vi "PAT Device Software 1.6.vi"() -> ()   [LabVIEW 2018]
uses:
  <vilib>/Utility/error.llb/DialogType.ctl
  <vilib>/DAQmx/write.llb/DAQmx Write (Analog 1D DBL NChan 1Samp).vi
  <vilib>/DAQmx/read.llb/DAQmx Read (Analog 1D DBL NChan 1Samp).vi
  <vilib>/DAQmx/write.llb/DAQmx Write (Analog DBL 1Chan 1Samp).vi
  <vilib>/Instr/_visa.llb/VISA Configure Serial Port (Instr).vi
  <vilib>/DAQmx/create/channels.llb/DAQmx Create Channel (AO-Voltage-Basic).vi
  <vilib>/DAQmx/create/channels.llb/DAQmx Create Channel (AI-Voltage-Basic).vi
  <vilib>/DAQmx/configure/timing.llb/DAQmx Timing (Sample Clock).vi
  <vilib>/DAQmx/miscellaneous.llb/DAQmx Fill In Error Info.vi
panel:
  out "Load Preset":bool
  in  "command line":string="cmd /c \"C:\\Program Files (x86)\\QTenki\\usbtenkiget.exe\" -s E13367 -i 0,1,2"
  in  "Test Length":i32=15
  in  "Minute Volume":dbl format="%#_13g"
  out "CV2 Voltage":dbl format="%#_13g"
  out "CV1 Voltage":dbl format="%#_13g"
  in  "In Progress":bool
  out "Total Test Time":i32
  in  "Test Buffer Duration":i32=10
  in  "Motor Control":bool
  out "Corrected Voltage":dbl=3.0 format="%#_13g"
  out "Rotation Time":dbl format="%#_3g"
  out "Error Ratio":dbl format="%#_13g"
  out "Reference Voltage":dbl=3.001413381851861 format="%0.2f"
  out "Hit Recorded":bool
  in  "CV2 Output":tag="Dev1/ao0"
  in  "CV1 Output":tag="Dev1/ao1"
  in  "Motor Output":tag="Dev2/ao0"
  in  "Hall Sensor Channel":tag="Dev2/ai7"
  in  "O2 Channel":tag="Dev2/ai6"
  in  "P2 Channel":tag="Dev2/ai4"
  in  "Relay Port":refnum<visa-resource-name>="COM13"
  in  "Sample Rate":i32=10
  in  "CV2 Channel":tag="Dev1/ai6"
  in  "CV1 Channel":tag="Dev1/ai3"
  in  "P1 Channel":tag="Dev1/ai5"
  out "Stop Test":bool=TRUE
  out "Is PAT Test?":bool
  in  "Test Begin":bool
  out "Test Duration":i32
  out "Current Test":string
  out "Test Underway":i32
  out "Number of tests":i32=4
  out "Test List":i16[](array[numeric])=[1, 1, 1, 1, 0, 0]
  out "error out 3":errorcluster
  in  "error in 2":errorcluster
  out "error out 2":errorcluster
  in  "error in":errorcluster
  out "error out":errorcluster
  in  "error in (no error)":errorcluster
  in  "Tab Control":enum32{"PAT Test", "Manual Control"}(tab)
  out "PAT Test Readings":T1 {"B40 S" scale=0.0..100.0; "B15 S" scale=0.0..100.0; "Ex70 S" scale=0.0..100.0; "Ex30 S" scale=0.0..100.0; "In70 S" scale=0.0..100.0; "B15 M" format="%#.2g"; "B40 M" format="%#.2g"; "Ex70 M" format="%#.2g"; "Ex30 M" format="%#.2g"; "In70 M" format="%#.2g"; "In30 S" scale=0.0..100.0; "In30 M" format="%#.2g"}
  out "Status":string="Status"
  out "Time":string="Time (s)"
  out "Limit":string="Limit"
  out "Comp":string="Comp"
  out "Units":string="Units"
  out "Measured":string="Measured"
  out "Test Name":string="Test Name"
  out "String 22":string="-0.8"
  out "String 24":string="0.8"
  out "String 23":string="-2.0"
  out "String 26":string="26"
  out "String 25":string="2.0"
  out "String 27":string="89"
  out "String 15":string=">="
  out "String 17":string="<="
  out "String 16":string=">="
  out "String 19":string=">="
  out "String 18":string="<="
  out "String 20":string=">="
  out "In H2O":string="in H2O"
  out "In H2O":string="in H2O"
  out "In H2O":string="in H2O"
  out "%O2":string="% O2"
  out "In H2O":string="in H2O"
  out "%O2":string="% O2"
  out "Inhalation 30lpm":string="Inhalation (30lpm)"
  out "Exhalation 30lpm":string="Exhalation (30lpm)"
  out "Inhalation 70lpm":string="Inhalation (70lpm)"
  out "Breathing 15kft":string="Breathing (15kft)"
  out "Exhalation 70lpm":string="Exhalation (70lpm)"
  out "Breathing 40kft":string="Breathing (40kft)"
  in  "Start PAT Test":bool
  in  "Stop PAT Test":bool
  out "Test Status:":string
  in  "Results File Location:":path=path "C:/"
  in  "PAT Test Fields":T2={"Operator:"="", "Pull Test Date:"="", "Manufacture Date:"="", "Cure Date:"="", "Production Order No.:"="", "Production Lot:"="", "No. Masks in Lot:"="", "Comments:"="", "Test Date:"="24 Jan 2019", "Test Time:"="11:23:54", "Test Selection Radio Array"=[TRUE, TRUE, TRUE, TRUE, FALSE, FALSE], "Test Parameters:"=enum."Quick Test", "F2 Leakage"=0.0}
  out "Ambient Pressure:":dbl format="%#.2g"
  out "Ambient Temp.:":dbl format="%#.2g"
  out "Ambient Humidity:":dbl format="%#.2g"
  in  "Preset Directory:":path=path "C:/"
  in  "MC Fields":T3={"Test Date:"="24 Jan 2019", "Test Time:"="11:23:54", "Operator:"="", "Production Order No.:"="", "Production Lot:"="", "No. Masks in Lot:"="", "Test Duration"=0, "Presets in Directory:"=0, "MC Test Length"=enum."Run Continuously", "Current Preset:"="Breathing Test 2.ini", "Preset Save"=FALSE}
  in  "MC Instrumentation":T4={"SV1"=FALSE, "SV2"=FALSE, "SV3"=FALSE, "SV4"=FALSE, "SV5"=FALSE, "SV6"=FALSE, "SV7"=FALSE, "SV8"=FALSE, "SV9"=FALSE, "M1"=FALSE, "MP1"=FALSE, "MP2"=FALSE, "CV1"=FALSE, "CV2"=FALSE, "CV1 Flow Rate:"=0.0, "CV2 Flow Rate:"=0.0, "P2 Pressure:"=0.0, "O2 Concentration:"=0.0, "Motor Speed:"=15.0, "F2 Leakage"=0.0, "P1 Pressure:"=0.0} {"P1 Pressure:" format="%#.2g"; "P2 Pressure:" format="%#.2g"; "O2 Concentration:" format="%#.2g"; "Motor Speed:" min=0.0 max=17.5 step=0.25 format="%#.2g"; "F2 Leakage" min=0.0 max=100.0 step=1.0; "CV2 Flow Rate:" min=0.0 max=100.0 format="%#.2g"; "CV1 Flow Rate:" min=0.0 max=5.0 step=0.5}
  in  "Start Custom Test":bool
  in  "Stop Custom Test":bool
  # "ccm"
  # "s"
  # "Pamb"
  # "Tamb"
  # "Hamb"
  # "in H2O"
  # "°C"
  # "%"
  # "O2"
  # "P"
  # "P"
  # "O2 Supply"
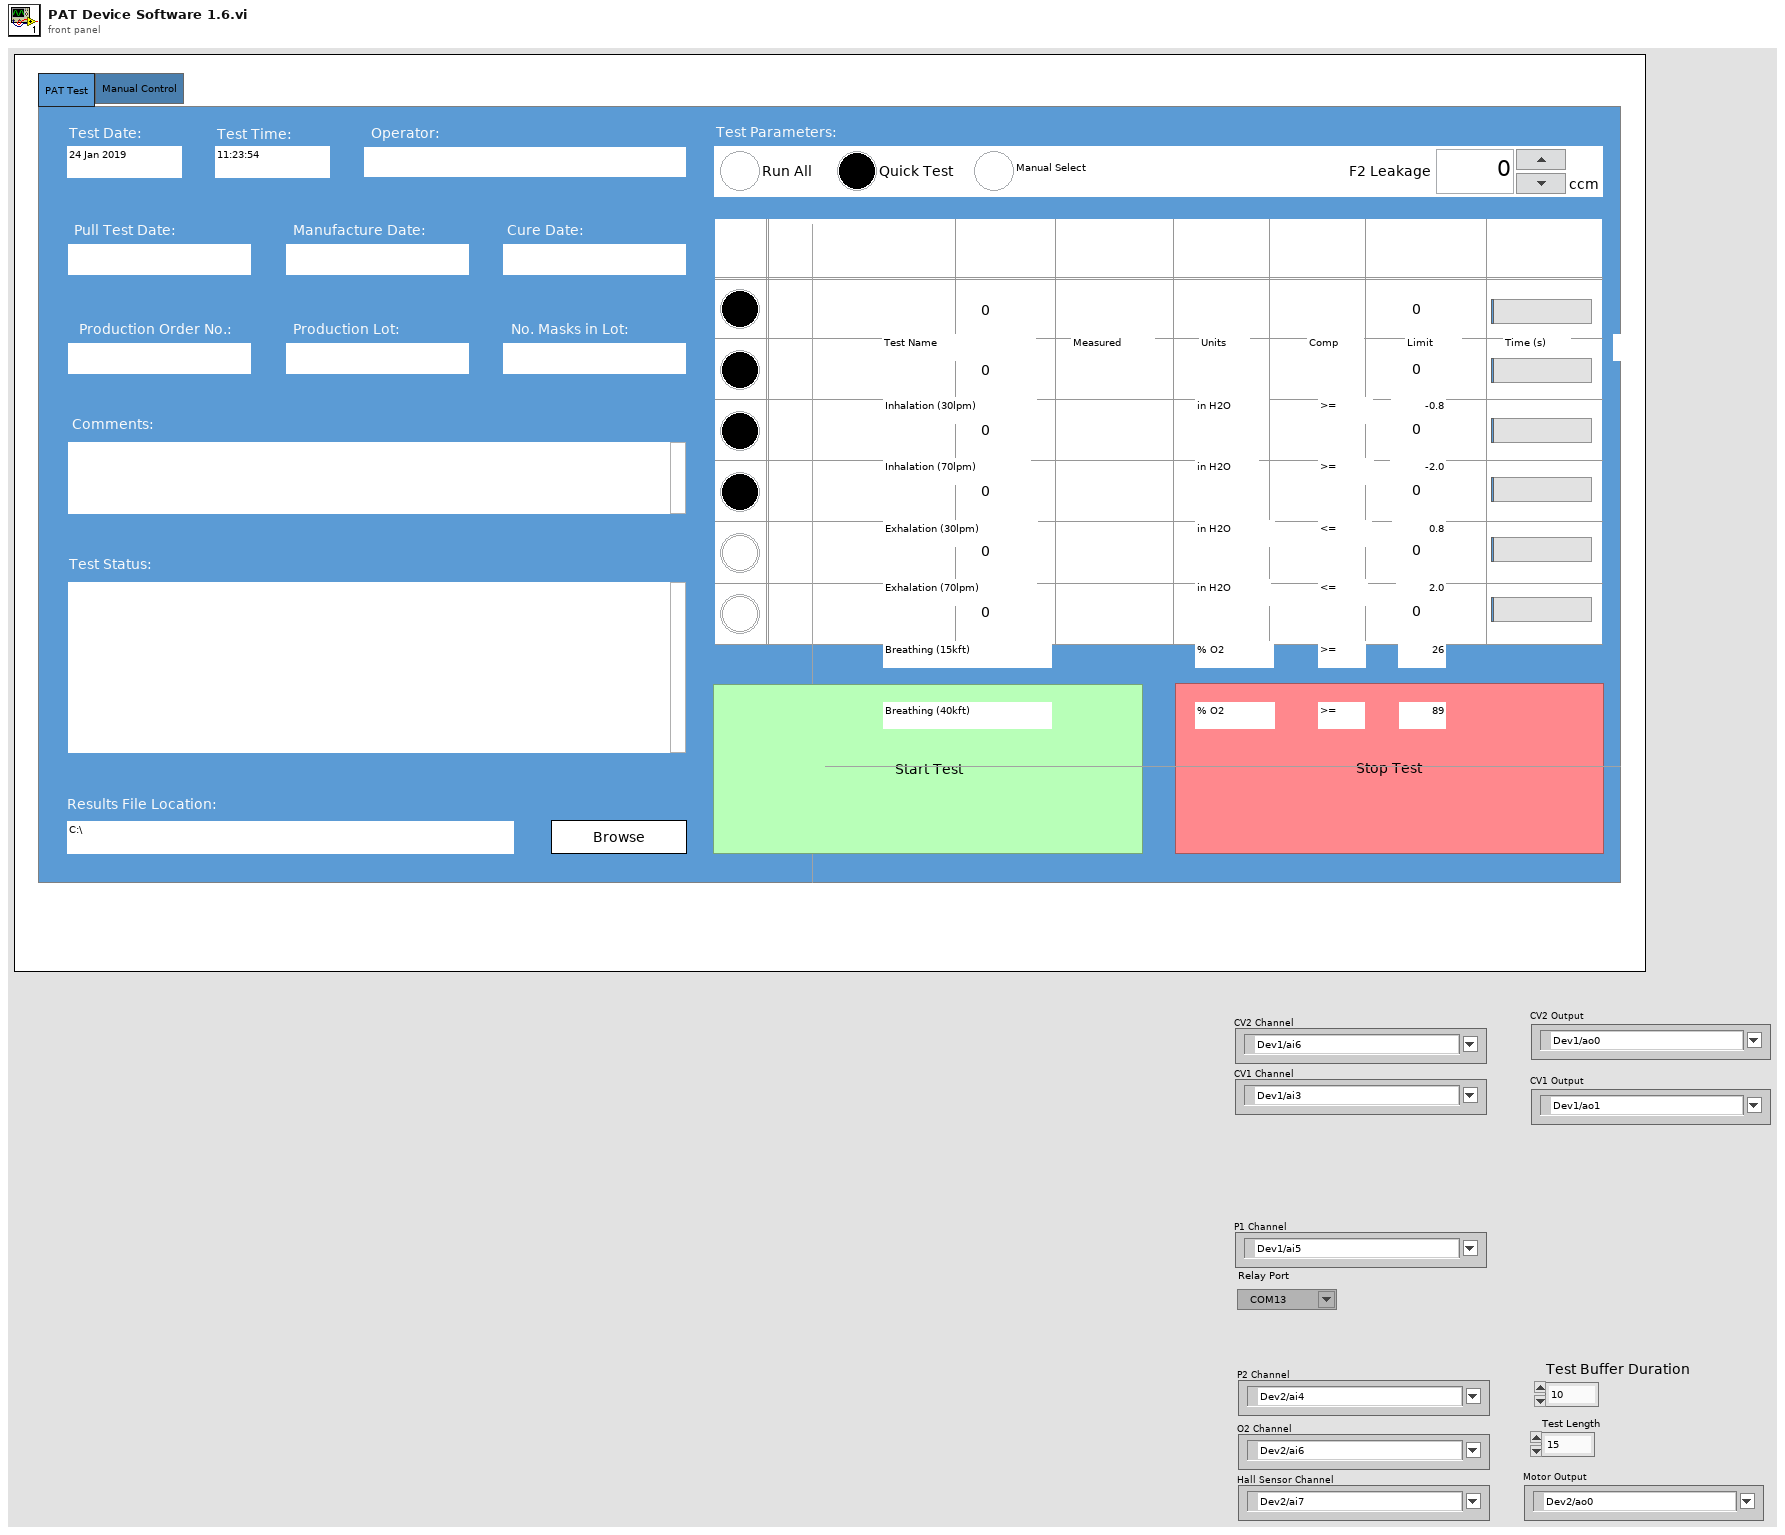
[diagram p1: front panel]
types:
  T1 = cluster{"In30 M":dbl, "In30 T":i64, "In30 S":u8, "In70 M":dbl, "Ex30 M":dbl, "Ex70 M":dbl, "B40 M":dbl, "B15 M":dbl, "In70 T":i64, "Ex30 T":i64, "Ex70 T":i64, "B40 T":i64, "B15 T":i64, "In70 S":u8, "Ex30 S":u8, "Ex70 S":u8, "B15 S":u8, "B40 S":u8}
  T2 = cluster{"Operator:":string, "Pull Test Date:":string, "Manufacture Date:":string, "Cure Date:":string, "Production Order No.:":string, "Production Lot:":string, "No. Masks in Lot:":string, "Comments:":string, "Test Date:":string, "Test Time:":string, "Test Selection Radio Array":bool[], "Test Parameters:":enum32{"Run All", "Quick Test", "Manual Select"}, "F2 Leakage":dbl}
  T3 = cluster{"Test Date:":string, "Test Time:":string, "Operator:":string, "Production Order No.:":string, "Production Lot:":string, "No. Masks in Lot:":string, "Test Duration":i64, "Presets in Directory:":i32, "MC Test Length":enum32{"Run Continuously", "Run for:"}, "Current Preset:":string, "Preset Save":bool}
  T4 = cluster{"SV1":bool, "SV2":bool, "SV3":bool, "SV4":bool, "SV5":bool, "SV6":bool, "SV7":bool, "SV8":bool, "SV9":bool, "M1":bool, "MP1":bool, "MP2":bool, "CV1":bool, "CV2":bool, "CV1 Flow Rate:":dbl, "CV2 Flow Rate:":dbl, "P2 Pressure:":dbl, "O2 Concentration:":dbl, "Motor Speed:":dbl, "F2 Leakage":dbl, "P1 Pressure:":dbl}
  T5 = enum8{"Enabled", "Disabled", "Disabled and Grayed Out"}
  T6 = typedef "DialogType.ctl" = u16
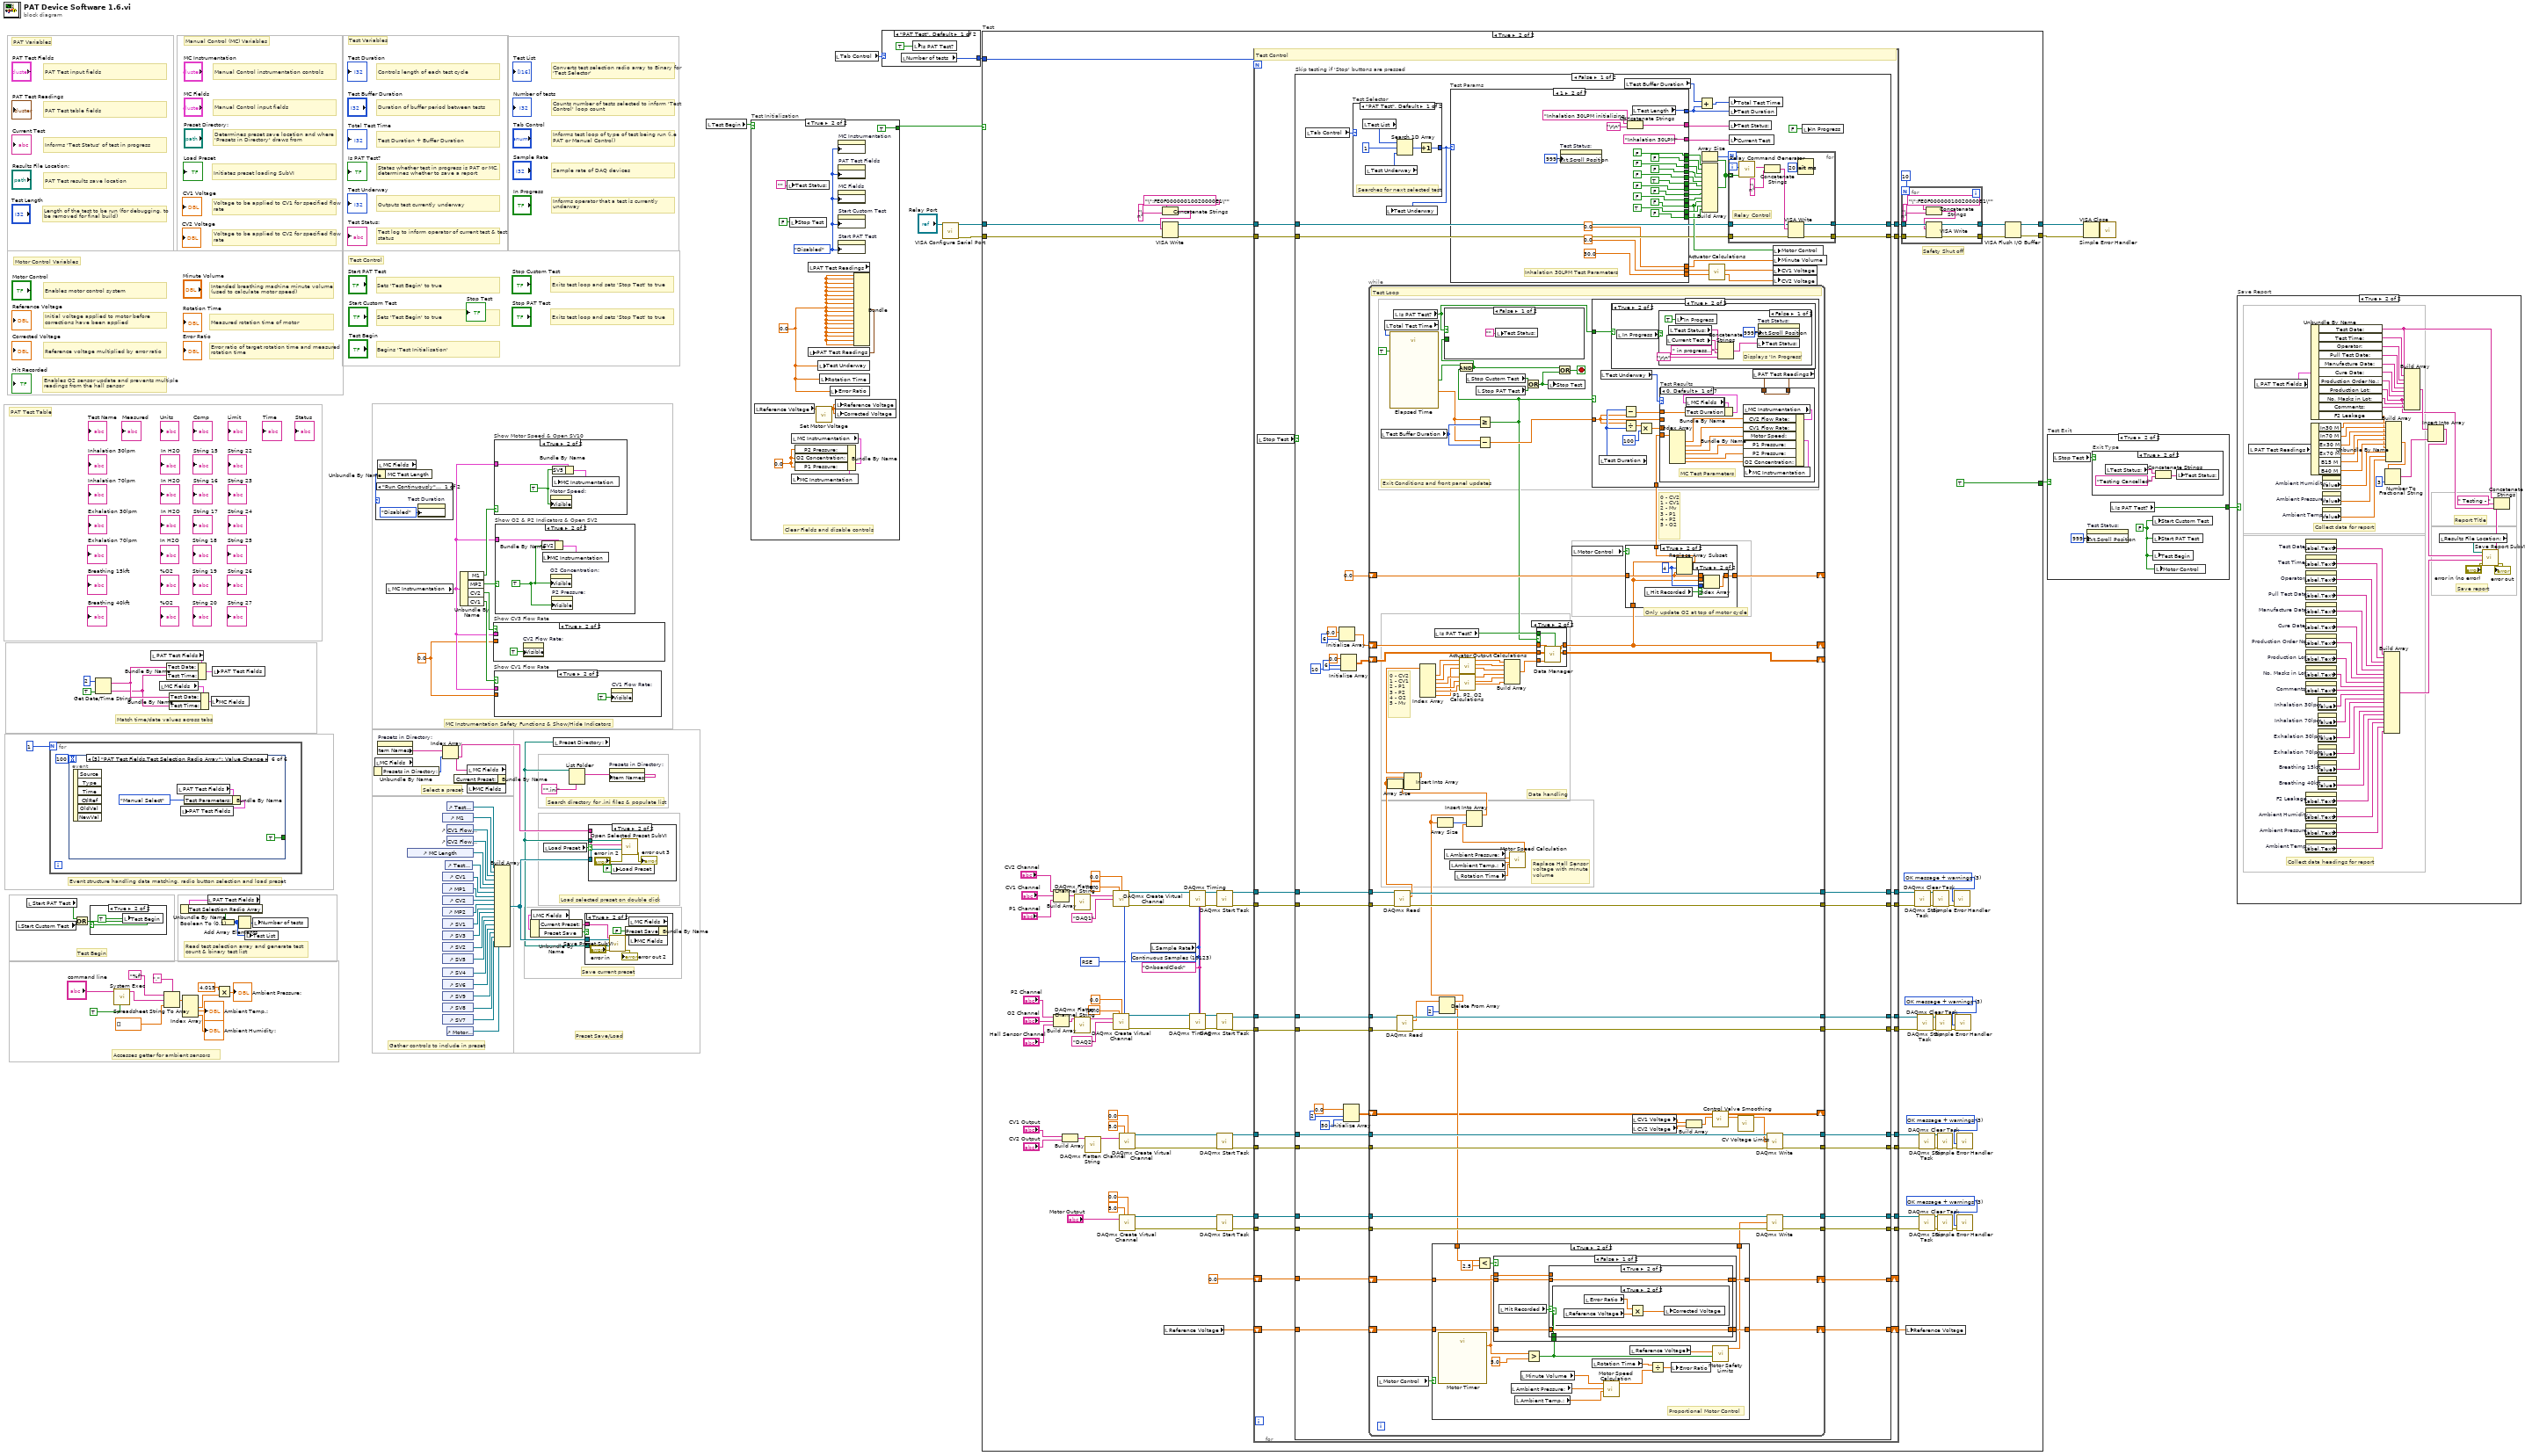
[diagram p0: block diagram]
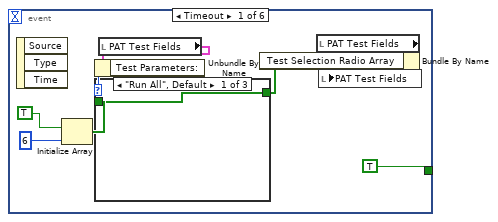
[diagram p2: hidden frame]
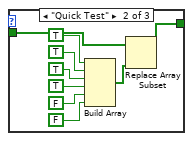
[diagram p3: hidden frame]
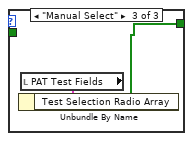
[diagram p4: hidden frame]
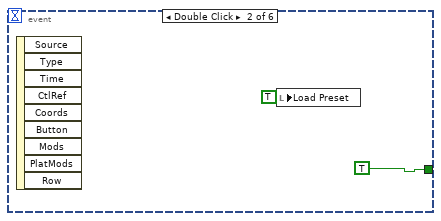
[diagram p5: hidden frame]
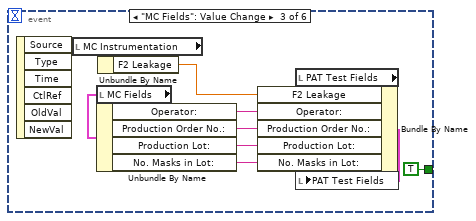
[diagram p6: hidden frame]
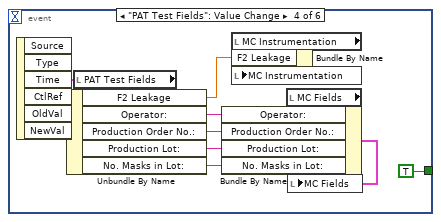
[diagram p7: hidden frame]
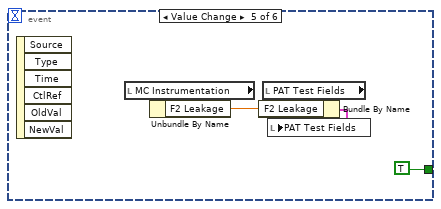
[diagram p8: hidden frame]
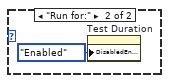
[diagram p11: hidden frame]
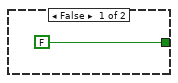
[diagram p12: hidden frame]
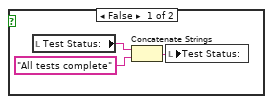
[diagram p13: hidden frame]
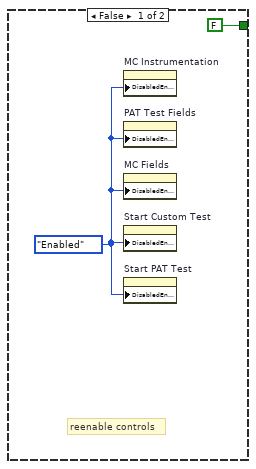
[diagram p14: hidden frame]
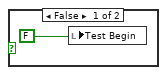
[diagram p15: hidden frame]
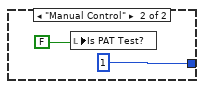
[diagram p16: hidden frame]
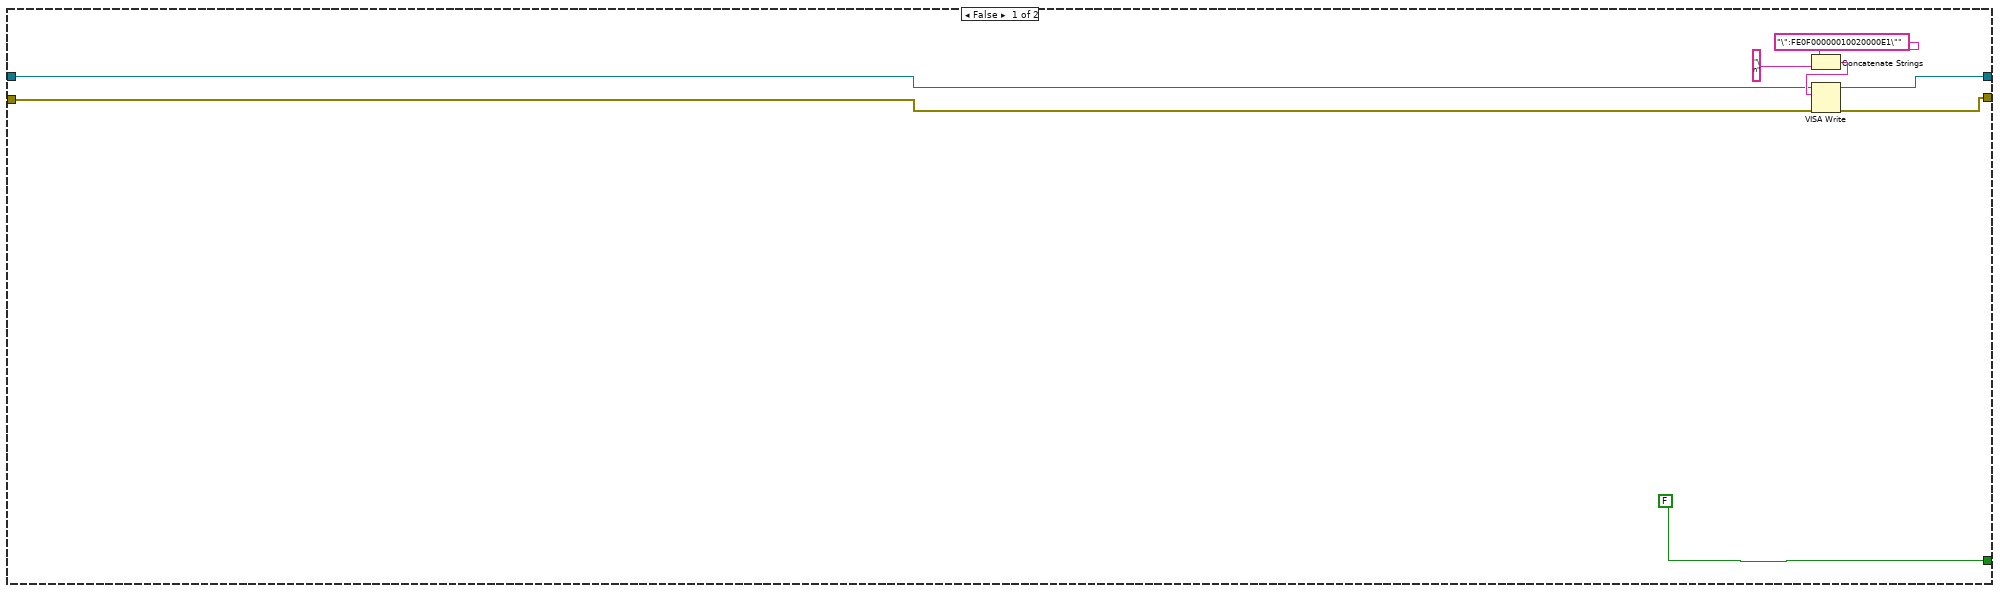
[diagram p17: hidden frame]
diagram:
  w27 = 0.0
  # "Length of the test to be run (for debugging, to be removed for final build)"
  # "Voltage to be applied to CV2 for specified flow rate"
  # "Voltage to be applied to CV1 for specified flow rate"
  # "Initiates preset loading SubVI"
  # "Accesses getter for ambient sensors"
  # "Enables O2 sensor update and prevents multiple readings from the hall sensor"
  # "Error ratio of target rotation time and measured rotation time"
  # "Measured rotation time of motor"
  # "Intended breathing machine minute volume (used to calculate motor speed)"
  # "Reference voltage multiplied by error ratio"
  # "Initial voltage applied to motor before corrections have been applied"
  # "Enables motor control system"
  # "Motor Control Variables"
  # "Informs operator that a test is currently underway"
  # "Sample rate of DAQ devices"
  # "Test log to inform operator of current test & test status"
  # "Outputs test currently underway"
  # "Test Duration + Buffer Duration"
  # "Duration of buffer period between tests"
  # "Preset Save/Load"
  # "Save current preset"
  # "Load selected preset on double click"
  # "Search directory for .ini files & populate list"
  # "Gather controls to include in preset"
  # "Select a preset"
  # "Read test selection array and generate test count & binary test list"
  # "MC Instrumentation Safety Functions & Show/Hide Indicators"
  # "Determines preset save location and where 'Presets in Directory' draws from"
  # "Test Control"
  # "Exits test loop and sets 'Stop Test' to true"
  # "Exits test loop and sets 'Stop Test' to true"
  # "Sets 'Test Begin' to true"
  # "Sets 'Test Begin' to true"
  # "PAT Test results save location"
  # "Informs test loop of type of test being run (i.e PAT or Manual Control)"
  # "Counts number of tests selected to inform 'Test Control' loop count"
  # "Begins 'Test Initialisation'"
  # "States whether test in progress is PAT or MC, determines whether to save a report"
  # "Controls length of each test cycle"
  # "Converts test selection radio array to Binary for 'Test Selector'"
  # "Test Begin"
  # "Test Variables"
  # "Manual Control input fields"
  # "Manual Control instrumentation controls"
  # "PAT Test input fields"
  # "PAT Test table fields"
  # "Informs 'Test Status' of test in progress"
  # "Manual Control (MC) Variables"
  # "Event structure handling data matching, radio button selection and load preset"
  # "Match time/date values across tabs"
  # "PAT Variables"
  # "PAT Test Table"
  n1 = local read "Start Custom Test"() -> (w41:bool)
  n2 = local read "Start PAT Test"() -> (w42:bool)
  n3 = for {
    N: 1 -> [_]
    n4 = event shown="[5] \"PAT Test Fields.Test Selection Radio Array\": Value Change" {
      selector: _ -> [_ _ _ _ _ _]
      dyn-events: _ -> [_ _ _ _ _ _]
      timeout: 100 -> [_ _ _ _ _ _]
      tunnel: [TRUE TRUE TRUE TRUE TRUE TRUE] -> _
      event Timeout {
        n5 = event-data() -> ()  [unwired: 1 in, 3 out]
        n6 = Initialize Array(TRUE, 6) -> (w87:bool[])
        n7 = local read "PAT Test Fields"() -> (w84:T2)
        n8 = Unbundle By Name(w84) -> ("Test Parameters:"=w91:enum32{"Run All", "Quick Test", "Manual Select"})
        n9 = case shown="\"Run All\", Default" w91 {
          tunnel: [w93 w96 w103] -> w90
          tunnel: w87 -> [w93 w94 _]
          frame "Run All", Default {
          }
          frame "Quick Test" {
            n10 = Build Array(TRUE, TRUE, TRUE, TRUE, FALSE, FALSE) -> (w95:bool[])
            n11 = Replace Array Subset(array=w94, new element=w95) -> (w96:bool[])  [unwired: 1 in]
          }
          frame "Manual Select" {
            n12 = local read "PAT Test Fields"() -> (w104:T2)
            n13 = Unbundle By Name(w104) -> ("Test Selection Radio Array"=w103:bool[])
          }
        }
        n14 = local read "PAT Test Fields"() -> (w88:T2)
        n15 = Bundle By Name(cluster=w88, "Test Selection Radio Array"=w90) -> (w89:T2)
        n16 = local write "PAT Test Fields"(w89) -> ()
      }
      event "MC Fields.Presets in Directory:": Double Click {
        n17 = event-data() -> ()  [unwired: 1 in, 9 out]
        n18 = local write "Load Preset"(TRUE ("Boolean")) -> ()
      }
      event "MC Fields": Value Change {
        n19 = event-data() -> ()  [unwired: 1 in, 6 out]
        n20 = local read "MC Instrumentation"() -> (w109:T4)
        n21 = local read "MC Fields"() -> (w108:T3)
        n22 = Unbundle By Name(w108) -> ("Operator:"=w112:string, "Production Order No.:"=w113:string, "Production Lot:"=w114:string, "No. Masks in Lot:"=w115:string)
        n23 = Unbundle By Name(w109) -> ("F2 Leakage"=w116:dbl)
        n24 = local read "PAT Test Fields"() -> (w110:T2)
        n25 = Bundle By Name(cluster=w110, "F2 Leakage"=w116, "Operator:"=w112, "Production Order No.:"=w113, "Production Lot:"=w114, "No. Masks in Lot:"=w115) -> (w111:T2)
        n26 = local write "PAT Test Fields"(w111) -> ()
      }
      event "PAT Test Fields": Value Change {
        n27 = event-data() -> ()  [unwired: 1 in, 6 out]
        n28 = local read "PAT Test Fields"() -> (w120:T2)
        n29 = Unbundle By Name(w120) -> ("F2 Leakage"=w121:dbl, "Operator:"=w124:string, "Production Order No.:"=w125:string, "Production Lot:"=w126:string, "No. Masks in Lot:"=w127:string)
        n30 = local read "MC Instrumentation"() -> (w119:T4)
        n31 = Bundle By Name(cluster=w119, "F2 Leakage"=w121) -> (w118:T4)
        n32 = local write "MC Instrumentation"(w118) -> ()
        n33 = local read "MC Fields"() -> (w122:T3)
        n34 = Bundle By Name(cluster=w122, "Operator:"=w124, "Production Order No.:"=w125, "Production Lot:"=w126, "No. Masks in Lot:"=w127) -> (w123:T3)
        n35 = local write "MC Fields"(w123) -> ()
      }
      event "MC Instrumentation.F2 Leakage": Value Change {
        n36 = event-data() -> ()  [unwired: 1 in, 6 out]
        n37 = local read "MC Instrumentation"() -> (w131:T4)
        n38 = Unbundle By Name(w131) -> ("F2 Leakage"=w132:dbl)
        n39 = local read "PAT Test Fields"() -> (w130:T2)
        n40 = Bundle By Name(cluster=w130, "F2 Leakage"=w132) -> (w129:T2)
        n41 = local write "PAT Test Fields"(w129) -> ()
      }
      event "PAT Test Fields.Test Selection Radio Array": Value Change {
        n42 = event-data() -> ()  [unwired: 1 in, 6 out]
        n43 = local read "PAT Test Fields"() -> (w135:T2)
        n44 = Bundle By Name(cluster=w135, "Test Parameters:"=enum32{"Run All", "Quick Test", "Manual Select"}."Manual Select") -> (w136:T2)
        n45 = local write "PAT Test Fields"(w136) -> ()
      }
    }
  }
  n46 = Or(x=w42, y=w41) -> (x .or. y?=w47:bool)
  n47 = case shown="True" w47 {
    frame False {
      n48 = local write "Test Begin"(FALSE) -> ()
    }
    frame True {
      n49 = local write "Test Begin"(TRUE) -> ()
    }
  }
  n50 = Get Date/Time String(date format (0)=2, want seconds? (F)=TRUE) -> (date string=w49:string, time string=w48:string)  [unwired: 1 in]
  n51 = call <vilib>:"System Exec.vi"("run minimized? (F)"=TRUE, "command line"="command line") -> ("standard output"=w15:string)  [unwired: 6 in, 3 out]
  n52 = local read "PAT Test Fields"() -> (w61:T2)
  n53 = local read "MC Fields"() -> (w55:T3)
  n54 = Spreadsheet String To Array(delimiter (Tab)=",", format string="%f", spreadsheet string=w15, array type (2D Dbl)=dbl[] []) -> (array=w17:dbl[])
  n55 = Bundle By Name(cluster=w61, "Test Date:"=w49, "Test Time:"=w48) -> (w60:T2)
  n56 = Bundle By Name(cluster=w55, "Test Date:"=w49, "Test Time:"=w48) -> (w54:T3)
  n57 = Index Array(array=w17) -> (element #1=w6:dbl, element #2=→"Ambient Temp.:":dbl, element #3=→"Ambient Humidity:":dbl)  [unwired: 3 in]
  n58 = local read "PAT Test Fields"() -> (w46:T2)
  n59 = Unbundle By Name(w46) -> ("Test Selection Radio Array"=w57:bool[])
  n60 = local write "MC Fields"(w54) -> ()
  n61 = local write "PAT Test Fields"(w60) -> ()
  n62 = Multiply(x=4.019, y=w6) -> (x*y=→"Ambient Pressure:":dbl)
  n63 = Boolean To (0,1)(Boolean=w57) -> (0, 1=w44:i16[])
  n64 = Add Array Elements(numeric array=w44) -> (sum=w45:i16)
  n65 = local write "Test List"(w44) -> ()
  n66 = local write "Number of tests"(w45) -> ()
  n67 = local read "MC Fields"() -> (w51:T3)
  n68 = Unbundle By Name(w51) -> ("Presets in Directory:"=w50:i32)
  n69 = local read "MC Fields"() -> (w33:T3)
  n70 = Unbundle By Name(w33) -> ("MC Test Length"=w32:enum32{"Run Continuously", "Run for:"})
  n71 = case shown="\"Run Continuously\", Default" w32 {
    frame "Run Continuously", Default {
      n72 = property on="Test Duration" class="DigNum (strict)"("DisabledEnum"=T5."Disabled" ("Disabled")) -> ()  [unwired: 2 in, 2 out]
    }
    frame "Run for:" {
      n73 = property on="Test Duration" class="DigNum (strict)"("DisabledEnum"=T5."Enabled" ("Disabled")) -> ()  [unwired: 2 in, 2 out]
    }
  }
  n74 = property on="Presets in Directory:" class="LstBox (strict)"() -> ("Item Names"=w63:string[])  [unwired: 2 in, 2 out]
  n75 = local read "MC Instrumentation"() -> (w28:T4)
  n76 = control-ref of="MC Length"() -> (w53:refnum<vi>)
  n77 = Index Array(array=w63, index=w50) -> (element=w24:string)
  n78 = control-ref of="M1"() -> (w79:refnum<vi>)
  n79 = control-ref of="CV1"() -> (w31:refnum<vi>)
  n80 = control-ref of="MP1"() -> (w75:refnum<vi>)
  n81 = control-ref of="CV2"() -> (w76:refnum<vi>)
  n82 = control-ref of="MP2"() -> (w74:refnum<vi>)
  n83 = control-ref of="SV1"() -> (w73:refnum<vi>)
  n84 = control-ref of="SV3"() -> (w72:refnum<vi>)
  n85 = control-ref of="SV2"() -> (w71:refnum<vi>)
  n86 = control-ref of="SV5"() -> (w70:refnum<vi>)
  n87 = control-ref of="SV4"() -> (w69:refnum<vi>)
  n88 = control-ref of="SV6"() -> (w68:refnum<vi>)
  n89 = control-ref of="SV9"() -> (w67:refnum<vi>)
  n90 = control-ref of="SV8"() -> (w66:refnum<vi>)
  n91 = control-ref of="SV7"() -> (w65:refnum<vi>)
  n92 = control-ref of="Test Duration"() -> (w52:refnum<vi>)
  n93 = control-ref of="Test Duration"() -> (w80:refnum<vi>)
  n94 = control-ref of="CV1 Flow Rate:"() -> (w78:refnum<vi>)
  n95 = control-ref of="CV2 Flow Rate:"() -> (w77:refnum<vi>)
  n96 = control-ref of="Motor Speed:"() -> (w18:refnum<vi>)
  n97 = Unbundle By Name(w28) -> ("M1"=w58:bool, "MP2"=w30:bool, "CV2"=w29:bool, "CV1"=w59:bool)
  n98 = local read "MC Fields"() -> (w36:T3)
  n99 = Bundle By Name(cluster=w36, "Current Preset:"=w24) -> (w35:T3)
  n100 = local write "MC Fields"(w35) -> ()
  n101 = case "Show CV3 Flow Rate" shown="True" w29 {
    tunnel: w28 -> [w143 _]
    tunnel: w27 -> [w141 _]
    frame False {
      n102 = Bundle By Name(cluster=w143, "CV2 Flow Rate:"=w141) -> (w144:T4)
      n103 = local write "MC Instrumentation"(w144) -> ()
      n104 = property on="CV2 Flow Rate:" class="DigNum (strict)"("Visible"=FALSE) -> ()  [unwired: 2 in, 2 out]
    }
    frame True {
      n105 = property on="CV2 Flow Rate:" class="DigNum (strict)"("Visible"=TRUE) -> ()  [unwired: 2 in, 2 out]
    }
  }
  n106 = case "Show Motor Speed & Open SV10" shown="True" w58 {
    tunnel: w28 -> [_ w148]
    frame False {
      n107 = property on="Motor Speed:" class="DigNum (strict)"("Visible"=FALSE) -> ()  [unwired: 2 in, 2 out]
    }
    frame True {
      w149 = TRUE ("Visible")
      n108 = property on="Motor Speed:" class="DigNum (strict)"("Visible"=w149) -> ()  [unwired: 2 in, 2 out]
      n109 = Bundle By Name(cluster=w148, "SV5"=w149) -> (w147:T4)
      n110 = local write "MC Instrumentation"(w147) -> ()
    }
  }
  n111 = case "Show CV1 Flow Rate" shown="True" w59 {
    tunnel: w28 -> [w152 _]
    tunnel: w27 -> [w150 _]
    frame False {
      n112 = Bundle By Name(cluster=w152, "CV1 Flow Rate:"=w150) -> (w151:T4)
      n113 = local write "MC Instrumentation"(w151) -> ()
      n114 = property on="CV1 Flow Rate:" class="DigNum (strict)"("Visible"=FALSE) -> ()  [unwired: 2 in, 2 out]
    }
    frame True {
      n115 = property on="CV1 Flow Rate:" class="DigNum (strict)"("Visible"=TRUE) -> ()  [unwired: 2 in, 2 out]
    }
  }
  n116 = Build Array(w80, w79, w78, w77, w53, w52, w31, w75, w76, w74, w73, w72, w71, w70, w69, w68, w67, w66, w65, w18) -> (w25:refnum<vi>[])
  n117 = case "Show O2 & P2 Indicators & Open SV2" shown="True" w30 {
    tunnel: w28 -> [_ w157]
    frame False {
      w155 = FALSE ("Visible")
      n118 = property on="O2 Concentration:" class="DigNum (strict)"("Visible"=w155) -> ()  [unwired: 2 in, 2 out]
      n119 = property on="P2 Pressure:" class="DigNum (strict)"("Visible"=w155) -> ()  [unwired: 2 in, 2 out]
    }
    frame True {
      w156 = TRUE ("Visible")
      n120 = Bundle By Name(cluster=w157, "SV2"=w156) -> (w158:T4)
      n121 = local write "MC Instrumentation"(w158) -> ()
      n122 = property on="O2 Concentration:" class="DigNum (strict)"("Visible"=w156) -> ()  [unwired: 2 in, 2 out]
      n123 = property on="P2 Pressure:" class="DigNum (strict)"("Visible"=w156) -> ()  [unwired: 2 in, 2 out]
    }
  }
  n124 = local read "MC Fields"() -> (w34:T3)
  n125 = Unbundle By Name(w34) -> ("Current Preset:"=w20:string, "Preset Save"=w21:bool)
  n126 = local read "Load Preset"() -> (w22:bool)
  n127 = local read "Preset Directory:"() -> (w23:path)
  n128 = List Folder(path=w23, pattern="*.ini") -> (filenames=w62:string[])  [unwired: 2 in, 3 out]
  n129 = case shown="True" w21 {
    tunnel: w20 -> [_ w166]
    tunnel: w25 -> [_ w165]
    tunnel: w23 -> [_ w164]
    frame False {
    }
    frame True {
      n130 = call "Save Preset SubVI.vi"("Control Settings"=w165, "error in (no error)"="error in", "Preset Directory:"=w164, "Preset Name"=w166) -> ("error out"=→"error out 2":errorcluster)  [unwired: 7 in]
      n131 = local read "MC Fields"() -> (w161:T3)
      n132 = Bundle By Name(cluster=w161, "Preset Save"=FALSE) -> (w160:T3)
      n133 = local write "MC Fields"(w160) -> ()
    }
  }
  n134 = case shown="True" w22 {
    tunnel: w25 -> [_ w171]
    tunnel: w24 -> [_ w170]
    tunnel: w23 -> [_ w169]
    frame False {
    }
    frame True {
      n135 = local write "Load Preset"(FALSE ("Boolean")) -> ()
      n136 = call "Open Selected Preset SubVI.vi"("error in (no error)"="error in 2", "Controls"=w171, "Current Preset"=w170, "Preset Directory:"=w169) -> ("error out"=→"error out 3":errorcluster)  [unwired: 7 in]
    }
  }
  n137 = property on="Presets in Directory:" class="LstBox (strict)"("Item Names"=w62) -> ()  [unwired: 2 in, 2 out]
  n138 = local read "Test Begin"() -> (w40:bool)
  n139 = case "Test Initialisation" shown="True" w40 {
    tunnel: [FALSE TRUE] -> w38
    frame False {
      w173 = T5."Enabled" ("Disabled")
      # "reenable controls"
      n140 = property on="MC Instrumentation" class="Clust (strict)"("DisabledEnum"=w173) -> ()  [unwired: 2 in, 2 out]
      n141 = property on="PAT Test Fields" class="Clust (strict)"("DisabledEnum"=w173) -> ()  [unwired: 2 in, 2 out]
      n142 = property on="MC Fields" class="Clust (strict)"("DisabledEnum"=w173) -> ()  [unwired: 2 in, 2 out]
      n143 = property on="Start Custom Test" class="Bool (strict)"("DisabledEnum"=w173) -> ()  [unwired: 2 in, 2 out]
      n144 = property on="Start PAT Test" class="Bool (strict)"("DisabledEnum"=w173) -> ()  [unwired: 2 in, 2 out]
    }
    frame True {
      w175 = 0.0
      w178 = 0.0
      w179 = T5."Disabled" ("Disabled")
      # "Clear Fields and disable controls"
      n145 = local read "Reference Voltage"() -> (w180:dbl)
      n146 = local write "Test Status:"("") -> ()
      n147 = local write "Stop Test"(FALSE ("Visible")) -> ()
      n148 = local read "MC Instrumentation"() -> (w177:T4)
      n149 = Bundle By Name(cluster=w177, "P2 Pressure:"=w175, "O2 Concentration:"=w175, "P1 Pressure:"=w175) -> (w176:T4)
      n150 = local write "MC Instrumentation"(w176) -> ()
      n151 = local read "PAT Test Readings"() -> (w186:T1)
      n152 = call "Set Motor Voltage.vi"("Reference Voltage in"=w180) -> ("Reference Voltage out"=w181:dbl)  [unwired: 10 in]
      n153 = local write "Test Underway"(w178) -> ()
      n154 = local write "Rotation Time"(w178) -> ()
      n155 = local write "Error Ratio"(w178) -> ()
      n156 = local write "Reference Voltage"(w181) -> ()
      n157 = local write "Corrected Voltage"(w181) -> ()
      n158 = property on="MC Instrumentation" class="Clust (strict)"("DisabledEnum"=w179) -> ()  [unwired: 2 in, 2 out]
      n159 = property on="PAT Test Fields" class="Clust (strict)"("DisabledEnum"=w179) -> ()  [unwired: 2 in, 2 out]
      n160 = property on="MC Fields" class="Clust (strict)"("DisabledEnum"=w179) -> ()  [unwired: 2 in, 2 out]
      n161 = property on="Start Custom Test" class="Bool (strict)"("DisabledEnum"=w179) -> ()  [unwired: 2 in, 2 out]
      n162 = property on="Start PAT Test" class="Bool (strict)"("DisabledEnum"=w179) -> ()  [unwired: 2 in, 2 out]
      n163 = Bundle(cluster=w186, "In30 M"=w178, "In30 T"=w178, "In30 S"=w178, "In70 M"=w178, "Ex30 M"=w178, "Ex70 M"=w178, "B40 M"=w178, "B15 M"=w178, "In70 T"=w178, "Ex30 T"=w178, "Ex70 T"=w178, "B40 T"=w178, "B15 T"=w178, "In70 S"=w178, "Ex30 S"=w178, "Ex70 S"=w178, "B15 S"=w178, "B40 S"=w178) -> (w185:T1)
      n164 = local write "PAT Test Readings"(w185) -> ()
    }
  }
  n165 = local read "Tab Control"() -> (w43:enum32{"PAT Test", "Manual Control"})
  n166 = case shown="\"PAT Test\", Default" w43 {
    tunnel: [w188 1] -> w56
    frame "PAT Test", Default {
      n167 = local read "Number of tests"() -> (w188:i32)
      n168 = local write "Is PAT Test?"(TRUE ("Boolean")) -> ()
    }
    frame "Manual Control" {
      n169 = local write "Is PAT Test?"(FALSE ("Boolean")) -> ()
    }
  }
  n170 = call-poly "VISA Configure Serial Port"("VISA resource name"="Relay Port") -> ("VISA resource name out"=w3:refnum<visa-resource-name>, "error out"=w2:errorcluster)  [unwired: 13 in]
  n171 = case "Test" shown="True" w38 {
    tunnel: w56 -> [_ w290]
    tunnel: [FALSE TRUE] -> w39
    tunnel: w3 -> [w192 w204]
    tunnel: w2 -> [w191 w205]
    tunnel: [w195 w209] -> w5
    tunnel: [w196 w210] -> w26
    frame False {
      n172 = Concatenate Strings("\":FE0F00000010020000E1\"" ("write buffer"), "\n" ("string")) -> (w194:string)
      n173 = VISA Write(VISA resource name=w192, write buffer=w194, error in (no error)=w191) -> (VISA resource name out=w196:refnum<visa-resource-name>, error out=w195:errorcluster)  [unwired: 1 out]
    }
    frame True {
      w221 = T6 3 items=["no dialog", "OK message", "continue or stop message", "OK message + warnings", "continue/stop + warnings"] ("type of dialog (OK msg:1)")
      w219 = 10083 items=["Default"=-1, "RSE"=10083, "NRSE"=10078, "Differential"=10106, "Pseudodifferential"=12529] ("input terminal configuration")
      w218 = tag "OnboardClock" ("source")
      w261 = T6 3 items=["no dialog", "OK message", "continue or stop message", "OK message + warnings", "continue/stop + warnings"] ("type of dialog (OK msg:1)")
      w262 = T6 3 items=["no dialog", "OK message", "continue or stop message", "OK message + warnings", "continue/stop + warnings"] ("type of dialog (OK msg:1)")
      w264 = T6 3 items=["no dialog", "OK message", "continue or stop message", "OK message + warnings", "continue/stop + warnings"] ("type of dialog (OK msg:1)")
      w216 = 10123 items=["Finite Samples"=10178, "Continuous Samples"=10123, "Hardware Timed Single Point"=12522] ("sample mode")
      # "Safety Shut off"
      n174 = Build Array("CV2 Channel", "CV1 Channel", "P1 Channel") -> (w275:tag[])
      n175 = Build Array("P2 Channel", "O2 Channel", "Hall Sensor Channel") -> (w233:tag[])
      n176 = Build Array("CV1 Output", "CV2 Output") -> (w253:tag[])
      n177 = call <vilib>:"DAQmx Flatten Channel String.vi"("names in"=w275) -> ("names out"=w276:string)  [unwired: 13 in, 1 out]
      n178 = call <vilib>:"DAQmx Flatten Channel String.vi"("names in"=w233) -> ("names out"=w241:string)  [unwired: 13 in, 1 out]
      n179 = call <vilib>:"DAQmx Flatten Channel String.vi"("names in"=w253) -> ("names out"=w246:string)  [unwired: 13 in, 1 out]
      n180 = call-poly <vilib>:"DAQmx Create Virtual Channel.vi"("maximum value"=5.0, "minimum value"=0.0, "input terminal configuration"=w219, "physical channels"=w276, "name to assign"="DAQ1") -> ("task out"=w287:refnum<k21>, "error out"=w288:errorcluster)  [unwired: 9 in]
      n181 = call-poly <vilib>:"DAQmx Create Virtual Channel.vi"("maximum value"=10.0, "minimum value"=0.0, "input terminal configuration"=w219, "physical channels"=w241, "name to assign"="DAQ2") -> ("task out"=w240:refnum<k21>, "error out"=w239:errorcluster)  [unwired: 9 in]
      n182 = call-poly <vilib>:"DAQmx Create Virtual Channel.vi"("maximum value"=5.0, "minimum value"=0.0, "physical channels"=w246) -> ("task out"=w256:refnum<k21>, "error out"=w257:errorcluster)  [unwired: 11 in]
      n183 = call-poly <vilib>:"DAQmx Create Virtual Channel.vi"("maximum value"=5.0, "minimum value"=0.0, "physical channels"="Motor Output") -> ("task out"=w226:refnum<k21>, "error out"=w225:errorcluster)  [unwired: 11 in]
      n184 = local read "Sample Rate"() -> (w217:i32)
      n185 = Concatenate Strings("\":FE0F00000010020000E1\"" ("write buffer"), "\n" ("string")) -> (w206:string)
      n186 = VISA Write(VISA resource name=w204, write buffer=w206, error in (no error)=w205) -> (VISA resource name out=w200:refnum<visa-resource-name>, error out=w201:errorcluster)  [unwired: 1 out]
      n187 = local read "Reference Voltage"() -> (w212:dbl)
      n188 = call-poly <vilib>:"DAQmx Timing.vi"("task/channels in"=w287, "sample mode"=w216, "rate"=w217, "source"=w218, "error in"=w288) -> ("task out"=w245:refnum<k21>, "error out"=w244:errorcluster)  [unwired: 9 in]
      n189 = call-poly <vilib>:"DAQmx Timing.vi"("task/channels in"=w240, "sample mode"=w216, "rate"=w217, "source"=w218, "error in"=w239) -> ("task out"=w242:refnum<k21>, "error out"=w243:errorcluster)  [unwired: 9 in]
      n190 = call <vilib>:"DAQmx Start Task.vi"("task/channels in"=w245, "error in"=w244) -> ("task out"=w279:refnum<k21>, "error out"=w280:errorcluster)  [unwired: 12 in]
      n191 = call <vilib>:"DAQmx Start Task.vi"("task/channels in"=w242, "error in"=w243) -> ("task out"=w235:refnum<k21>, "error out"=w234:errorcluster)  [unwired: 12 in]
      n192 = call <vilib>:"DAQmx Start Task.vi"("task/channels in"=w256, "error in"=w257) -> ("task out"=w250:refnum<k21>, "error out"=w249:errorcluster)  [unwired: 12 in]
      n193 = call <vilib>:"DAQmx Start Task.vi"("task/channels in"=w226, "error in"=w225) -> ("task out"=w229:refnum<k21>, "error out"=w230:errorcluster)  [unwired: 12 in]
      n194 = for {
        N: w290 -> [_]
        tunnel: w279 -> [w321]
        tunnel: w280 -> [w320]
        tunnel: [w319] -> w284
        tunnel: [w318] -> w283
        tunnel: [w316] -> w272
        tunnel: [w317] -> w271
        tunnel: [w315] -> w268
        tunnel: [w314] -> w267
        tunnel: w235 -> [w313]
        tunnel: w234 -> [w312]
        tunnel: w250 -> [w311]
        tunnel: w249 -> [w310]
        tunnel: [w309] -> w248
        tunnel: [w308] -> w247
        tunnel: w229 -> [w304]
        tunnel: w230 -> [w305]
        tunnel: [w306] -> w231
        tunnel: [w307] -> w232
        shift-right: [w301] -> _
        shift-left: 0.0 ("element") -> [w303]
        shift-right: [w300] -> w211
        shift-left: w212 -> [w302]
        tunnel: w201 -> [w299]
        tunnel: w200 -> [w298]
        # "Test Control"
        n195 = local read "Stop Test"() -> (w322:bool)
        n196 = case "Skip testing if 'Stop' buttons are pressed" shown="False" w322 {
          tunnel: w321 -> [w384 w787]
          tunnel: w320 -> [w383 w786]
          tunnel: [w382 w787] -> w319
          tunnel: [w381 w786] -> w318
          tunnel: [w364 w776] -> w316
          tunnel: [w363 w777] -> w317
          tunnel: [w362 w785] -> w315
          tunnel: [w361 w784] -> w314
          tunnel: w313 -> [w360 w785]
          tunnel: w312 -> [w359 w784]
          tunnel: w311 -> [w358 w783]
          tunnel: w310 -> [w357 w782]
          tunnel: [w356 w783] -> w309
          tunnel: [w355 w782] -> w308
          tunnel: w304 -> [w351 w781]
          tunnel: w305 -> [w352 w780]
          tunnel: [w353 w781] -> w306
          tunnel: [w354 w780] -> w307
          tunnel: w303 -> [w347 w779]
          tunnel: w302 -> [w346 w778]
          tunnel: [w345 w779] -> w301
          tunnel: [w344 w778] -> w300
          tunnel: w299 -> [w325 w776]
          tunnel: w298 -> [w324 w777]
          frame False {
            n197 = local read "Tab Control"() -> (w385:enum32{"PAT Test", "Manual Control"})
            n198 = Initialize Array(0.0 ("element"), 6 ("dimension size")) -> (w348:dbl[])
            n199 = Initialize Array(0.0 ("element"), 6 ("dimension size"), 10 ("dimension size")) -> (w326:dbl[][])
            n200 = Initialize Array(0.0, 2 ("dimension size"), 50 ("dimension size")) -> (w330:dbl[][])
            n201 = case "Test Selector" shown="\"PAT Test\", Default" w385 {
              tunnel: [w770 0] -> w380
              frame "PAT Test", Default {
                # "Searches for next selected test"
                n202 = local read "Test List"() -> (w771:i16[])
                n203 = local read "Test Underway"() -> (w772:i32)
                n204 = Search 1D Array(1D array=w771, element=1, start index (0)=w772) -> (index of element=w774:i32)
                n205 = Increment(x=w774) -> (x+1=w770:i32)
              }
              frame "Manual Control" {
              }
            }
            n206 = while {
              tunnel: w384 -> [w466]
              tunnel: w383 -> [w465]
              tunnel: [w463] -> w382
              tunnel: [w464] -> w381
              shift-right: [w400] -> _
              shift-left: w348 -> [w461]
              shift-right: [w399] -> _
              shift-left: w326 -> [w462]
              tunnel: [w459] -> w362
              tunnel: [w458] -> w361
              tunnel: w360 -> [w457]
              tunnel: w359 -> [w456]
              tunnel: w358 -> [w455]
              tunnel: w357 -> [w454]
              tunnel: [w453] -> w356
              tunnel: [w452] -> w355
              tunnel: w351 -> [w447]
              tunnel: w352 -> [w448]
              tunnel: [w449] -> w353
              tunnel: [w450] -> w354
              shift-right: [w444] -> w344
              shift-left: w346 -> [w442]
              shift-right: [w445] -> w345
              shift-left: w347 -> [w446]
              shift-right: [w429] -> _
              shift-left: 0.0 -> [w427]
              shift-right: [w409] -> _
              shift-left: w330 -> [w412]
              stop <- w471 stop-if-true
              # "0 - CV2\n1 - CV1\n2 - Mv\n3 - P1\n4 - P2\n5 - O2"
              # "Only update O2 at top of motor cycle"
              # "Data handling"
              # "0 - CV2\n1 - CV1\n2 - P1\n3 - P2\n4 - O2\n5 - Mv"
              # "Replace Hall Sensor \nvoltage with minute \nvolume"
              # "Exit Conditions and front panel updates"
              # "Test Loop"
              n207 = local read "Motor Control"() -> (w439:bool)
              n208 = local read "Test Buffer Duration"() -> (w438:i32)
              n209 = local read "Total Test Time"() -> (w470:i32)
              n210 = call "Elapsed Time"("Time Target (s)"=w470, "Auto Reset"=TRUE ("Reset")) -> ("Elapsed Time (s)"=w437:dbl, "Time has Elapsed"=w398:bool)  [unwired: 10 in, 6 out]
              n211 = local read "Is PAT Test?"() -> (w404:bool)
              n212 = call-poly <vilib>:"DAQmx Read.vi"("task/channels in"=w466, "error in"=w465) -> ("task out"=w463:refnum<k21>, "data"=w425:dbl[], "error out"=w464:errorcluster)  [unwired: 11 in]
              n213 = Array Size(array=w425) -> (size(s)=w451:i32)
              n214 = call-poly <vilib>:"DAQmx Read.vi"("task/channels in"=w457, "error in"=w456) -> ("task out"=w459:refnum<k21>, "data"=w441:dbl[], "error out"=w458:errorcluster)  [unwired: 11 in]
              n215 = local read "Is PAT Test?"() -> (w421:bool)
              n216 = Delete From Array(array=w441, index=2 ("dimension size")) -> (deleted portion=w426:dbl, array with subset deleted=w433:dbl[])  [unwired: 1 in]
              n217 = case shown="True" w439 {
                tunnel: w446 -> [w569 w581]
                tunnel: [w569 w580] -> w445
                tunnel: [w568 w579] -> w444
                tunnel: [0.0 ("element") w578] -> w443
                tunnel: w442 -> [w568 w577]
                tunnel: w426 -> [_ w575]
                frame False {
                }
                frame True {
                  # "Proportional Motor Control"
                  n218 = call "Motor Timer"() -> ("Elapsed Time (s)"=w576:dbl)  [unwired: 12 in, 7 out]
                  n219 = Less?(x=w575, y=2.5) -> (x < y?=w583:bool)
                  n220 = local read "Ambient Pressure:"() -> (w570:dbl)
                  n221 = local read "Ambient Temp.:"() -> (w571:dbl)
                  n222 = local read "Minute Volume"() -> (w573:dbl)
                  n223 = Greater?(x=w576, y=5.0) -> (0:w587:bool)
                  n224 = case shown="False" w583 {
                    tunnel: [w594 w607] -> w580
                    tunnel: w581 -> [w593 w607]
                    tunnel: w577 -> [w592 w606]
                    tunnel: [w591 w606] -> w579
                    tunnel: w587 -> [w589 _]
                    tunnel: w576 -> [w588 _]
                    frame False {
                      n225 = local read "Hit Recorded"() -> (w590:bool)
                      n226 = case shown="True" w590 {
                        tunnel: [w596 w602] -> w594
                        tunnel: w593 -> [w599 w602]
                        tunnel: w592 -> [_ w601]
                        tunnel: [w597 w601] -> w591
                        tunnel: w589 -> [_ w600]
                        tunnel: w588 -> [w596 _]
                        frame False {
                          n227 = Subtract(x=w596, y=w599) -> (x-y=w598:dbl)
                          n228 = local read "Corrected Voltage"() -> (w597:dbl)
                          n229 = local write "Rotation Time"(w598) -> ()
                          n230 = local write "Reference Voltage"(w597) -> ()
                          n231 = local write "Hit Recorded"(TRUE ("Boolean")) -> ()
                        }
                        frame True {
                          n232 = case shown="True" w600 {
                            frame False {
                            }
                            frame True {
                              n233 = local read "Reference Voltage"() -> (w604:dbl)
                              n234 = local read "Error Ratio"() -> (w603:dbl)
                              n235 = Multiply(x=w603, y=w604) -> (x*y=w605:dbl)
                              n236 = local write "Corrected Voltage"(w605) -> ()
                            }
                          }
                        }
                      }
                    }
                    frame True {
                      n237 = local write "Hit Recorded"(FALSE ("Counted")) -> ()
                    }
                  }
                  n238 = local read "Rotation Time"() -> (w584:dbl)
                  n239 = call "Motor Speed Calculation.vi"("Tamb"=w571, "Pamb"=w570, "Minute Volume (BTPS) In"=w573) -> ("Rotation Time Out"=w572:dbl)  [unwired: 7 in, 1 out]
                  n240 = local read "Reference Voltage"() -> (w574:dbl)
                  n241 = Divide(x=w584, y=w572) -> (x/y=w585:dbl)
                  n242 = local write "Error Ratio"(w585) -> ()
                  n243 = call "Motor Safety Limits.vi"("Reference Voltage in"=w574, "Boolean"=w587) -> ("Reference Voltage out"=w578:dbl)  [unwired: 9 in]
                }
              }
              n244 = Array Size(array=w433) -> (size(s)=w432:i32)
              n245 = local read "Ambient Pressure:"() -> (w401:dbl)
              n246 = local read "Ambient Temp.:"() -> (w402:dbl)
              n247 = local read "Rotation Time"() -> (w424:dbl)
              n248 = local read "Stop Custom Test"() -> (w468:bool)
              n249 = local read "Stop PAT Test"() -> (w467:bool)
              n250 = Greater Or Equal?(x=w437, y=w438) -> (x >= y?=w397:bool)
              n251 = And(x=w398, y=w397) -> (x .and. y?=w396:bool)
              n252 = case shown="False" w404 {
                tunnel: w396 -> [_ w610]
                frame False {
                  n253 = local write "Test Status:"("") -> ()
                }
                frame True {
                  n254 = case shown="True" w610 {
                    frame False {
                    }
                    frame True {
                      n255 = local read "Current Test"() -> (w613:string)
                      n256 = local read "Test Status:"() -> (w611:string)
                      n257 = Concatenate Strings(w611, w613, " complete", "\r\n") -> (w612:string)
                      n258 = local write "Test Status:"(w612) -> ()
                    }
                  }
                }
              }
              n259 = Subtract(x=w437, y=w438) -> (x-y=w436:dbl)
              n260 = call "Motor Speed Calculation.vi"("Rotation Time In"=w424, "Tamb"=w402, "Pamb"=w401) -> ("Minute Volume (BTPS) Out"=w423:dbl)  [unwired: 7 in, 1 out]
              n261 = Insert Into Array(array=w433, index=w432, new element=w423) -> (w431:dbl[])
              n262 = Insert Into Array(array=w425, index=w451, new element=w431) -> (w422:dbl[])
              n263 = Index Array(array=w422) -> (element #1=w420:dbl, element #2=w419:dbl, element #3=w408:dbl, element #4=w407:dbl, element #5=w406:dbl, element #6=w405:dbl)  [unwired: 6 in]
              n264 = call "Actuator Output Calculations.vi"("Minute Volume"=w405, "CV1 Voltage"=w419, "CV2 Voltage"=w420) -> ("Motor Speed"=w416:dbl, "CV1 Flow Rate"=w417:dbl, "CV2 Flow Rate"=w418:dbl)  [unwired: 6 in]
              n265 = call "P1, P2, O2 Calculations.vi"("O2 Voltage"=w406, "P2 Voltage"=w407, "P1 Voltage"=w408) -> ("O2"=w413:dbl, "P2 Pressure"=w414:dbl, "P1 Pressure"=w415:dbl)  [unwired: 6 in]
              n266 = Build Array(w418, w417, w416, w415, w414, w413) -> (w460:dbl[])
              n267 = Or(x=w468, y=w467) -> (x .or. y?=w469:bool)
              n268 = case shown="True" w397 {
                tunnel: w462 -> [w486 w492]
                tunnel: w461 -> [w485 w491]
                tunnel: w460 -> [_ w490]
                tunnel: [w486 w489] -> w399
                tunnel: [w485 w488] -> w400
                tunnel: w421 -> [_ w487]
                frame False {
                }
                frame True {
                  n269 = call "Data Manager.vi"("Max Av Values In"=w491, "Data Array In"=w492, "Data"=w490, "Is PAT Test?"=w487) -> ("Max Av Values Out"=w488:dbl[], "Data Array Out"=w489:dbl[][])  [unwired: 4 in]
                }
              }
              n270 = local write "Stop Test"(w469) -> ()
              n271 = Or(x=w396, y=w469) -> (x .or. y?=w471:bool)
              n272 = local read "Motor Control"() -> (w403:bool)
              n273 = case shown="True" w403 {
                tunnel: [w474 w478] -> w429
                tunnel: [w473 w477] -> w428
                tunnel: w427 -> [w474 w476]
                tunnel: w400 -> [w473 w475]
                frame False {
                }
                frame True {
                  w479 = 4 ("minimum value")
                  n274 = local read "Hit Recorded"() -> (w480:bool)
                  n275 = Replace Array Subset(array=w475, new element=w476, index=w479) -> (w477:dbl[])
                  n276 = case shown="True" w480 {
                    tunnel: w475 -> [_ w484]
                    tunnel: [w481 w483] -> w478
                    tunnel: w476 -> [w481 _]
                    tunnel: w479 -> [_ w482]
                    frame False {
                    }
                    frame True {
                      n277 = Index Array(array=w484, index=w482) -> (element=w483:dbl)
                    }
                  }
                }
              }
              n278 = case shown="True" w397 {
                tunnel: w428 -> [_ w497]
                tunnel: w436 -> [_ w494]
                tunnel: w404 -> [_ w496]
                frame False {
                }
                frame True {
                  n279 = local read "Test Duration"() -> (w495:i32)
                  n280 = local read "Test Underway"() -> (w503:i32)
                  n281 = case shown="True" w496 {
                    frame False {
                    }
                    frame True {
                      n282 = local read "In Progress"() -> (w504:bool)
                      n283 = case shown="False" w504 {
                        frame False {
                          # "Displays 'In Progress'"
                          n284 = local read "Current Test"() -> (w509:string)
                          n285 = local read "Test Status:"() -> (w511:string)
                          n286 = local write "In Progress"(TRUE ("Boolean 2")) -> ()
                          n287 = Concatenate Strings(w511, w509, " in progress...", "\r\n") -> (w510:string)
                          n288 = local write "Test Status:"(w510) -> ()
                          n289 = property on="Test Status:" class="Str"("Text.Scroll Position"=999) -> ()  [unwired: 2 in, 2 out]
                        }
                        frame True {
                        }
                      }
                    }
                  }
                  n290 = Subtract(x=w495, y=w494) -> (x-y=w493:dbl)
                  n291 = Divide(x=w494, y=w495) -> (x/y=w501:dbl)
                  n292 = Multiply(x=w501, y=100) -> (x*y=w499:dbl)
                  n293 = local read "PAT Test Readings"() -> (w502:T1)
                  n294 = case "Test Results" shown="0, Default" w503 {
                    tunnel: w494 -> [_ w529 w536 w543 w550 w557 w564]
                    tunnel: w502 -> [w523 w530 w537 w545 w552 w559 w565]
                    tunnel: w499 -> [_ w528 w535 w542 w549 w556 w563]
                    tunnel: [w523 w531 w538 w544 w551 w558 w566] -> w498
                    tunnel: w497 -> [w522 w527 w533 w540 w547 w554 w561]
                    tunnel: w493 -> [w512 _ _ _ _ _ _]
                    frame 0, Default {
                      # "MC Test Parameters"
                      n295 = Index Array(array=w522) -> (element #1=w520:dbl, element #2=w519:dbl, element #3=w518:dbl, element #4=w517:dbl, element #5=w516:dbl, element #6=w515:dbl)  [unwired: 6 in]
                      n296 = local read "MC Fields"() -> (w514:T3)
                      n297 = Bundle By Name(cluster=w514, "Test Duration"=w512) -> (w513:T3)
                      n298 = local write "MC Fields"(w513) -> ()
                      n299 = local read "MC Instrumentation"() -> (w521:T4)
                      n300 = Bundle By Name(cluster=w521, "CV2 Flow Rate:"=w520, "CV1 Flow Rate:"=w519, "Motor Speed:"=w518, "P1 Pressure:"=w517, "P2 Pressure:"=w516, "O2 Concentration:"=w515) -> (w524:T4)
                      n301 = local write "MC Instrumentation"(w524) -> ()
                    }
                    frame 1 {
                      # "Inhalation 30LPM Test Parameters"
                      n302 = Index Array(array=w527, index=3 ("minimum value")) -> (element=w525:dbl)
                      n303 = Bundle By Name(cluster=w530, "In30 T"=w529, "In30 S"=w528, "In30 M"=w525) -> (w531:T1)
                    }
                    frame 2 {
                      # "Inhalation 70LPM Test Parameters"
                      n304 = Index Array(array=w533, index=3 ("minimum value")) -> (element=w532:dbl)
                      n305 = Bundle By Name(cluster=w537, "In70 T"=w536, "In70 S"=w535, "In70 M"=w532) -> (w538:T1)
                    }
                    frame 3 {
                      # "Exhalation 30LPM Test Parameters"
                      n306 = Index Array(array=w540, index=3 ("minimum value")) -> (element=w539:dbl)
                      n307 = Bundle By Name(cluster=w545, "Ex30 T"=w543, "Ex30 S"=w542, "Ex30 M"=w539) -> (w544:T1)
                    }
                    frame 4 {
                      # "Exhalation 70LPM Test Parameters"
                      n308 = Index Array(array=w547, index=3 ("minimum value")) -> (element=w546:dbl)
                      n309 = Bundle By Name(cluster=w552, "Ex70 T"=w550, "Ex70 S"=w549, "Ex70 M"=w546) -> (w551:T1)
                    }
                    frame 5 {
                      # "Breathing 15kft Test Output"
                      n310 = Index Array(array=w554, index=5 ("minimum value")) -> (element=w553:dbl)
                      n311 = Bundle By Name(cluster=w559, "B15 T"=w557, "B15 S"=w556, "B15 M"=w553) -> (w558:T1)
                    }
                    frame 6 {
                      # "Breathing 40kft Test Output"
                      n312 = Index Array(array=w561, index=5 ("minimum value")) -> (element=w560:dbl)
                      n313 = Bundle By Name(cluster=w565, "B40 T"=w564, "B40 S"=w563, "B40 M"=w560) -> (w566:T1)
                    }
                  }
                  n314 = local write "PAT Test Readings"(w498) -> ()
                }
              }
              n315 = local read "CV1 Voltage"() -> (w435:dbl)
              n316 = local read "CV2 Voltage"() -> (w434:dbl)
              n317 = Build Array(w435, w434) -> (w411:dbl[])
              n318 = call "Control Valve Smoothing.vi"("CV Control Voltages"=w411, "Averaged In"=w412) -> ("Smoothed Voltage"=w410:dbl[], "Averaged Out"=w409:dbl[][])  [unwired: 8 in]
              n319 = call "CV Voltage Limits.vi"("CV Voltage In"=w410) -> ("CV Voltage Out"=w430:dbl[])  [unwired: 10 in]
              n320 = call-poly <vilib>:"DAQmx Write.vi"("task/channels in"=w455, "data"=w430, "error in"=w454) -> ("task out"=w453:refnum<k21>, "error out"=w452:errorcluster)  [unwired: 10 in, 1 out]
              n321 = call-poly <vilib>:"DAQmx Write.vi"("task/channels in"=w447, "data"=w443, "error in"=w448) -> ("task out"=w449:refnum<k21>, "error out"=w450:errorcluster)  [unwired: 10 in, 1 out]
            }
            n322 = local write "Test Underway"(w380) -> ()
            n323 = case "Test Params" shown="1" w380 {
              tunnel: [w631 w639 w660 w682 w704 w726 w748] -> w341
              tunnel: [w632 "Inhalation 30LPM" "Inhalation 70LPM" "Exhalation 30LPM" "Exhalation 70LPM" "Breathing 15kft" "Breathing 40kft"] -> w379
              tunnel: [w632 w655 w676 w698 w720 w742 w764] -> w378
              tunnel: [w630 FALSE FALSE FALSE FALSE TRUE TRUE] -> w377
              tunnel: [w629 FALSE ("element") FALSE ("element") FALSE ("element") FALSE ("element") TRUE ("element") TRUE ("element")] -> w376
              tunnel: [w628 FALSE ("element") FALSE ("element") FALSE ("element") FALSE ("element") TRUE ("element") TRUE ("element")] -> w375
              tunnel: [w627 FALSE ("element") FALSE ("element") FALSE ("element") FALSE ("element") FALSE ("element") FALSE ("element")] -> w374
              tunnel: [w620 FALSE ("element") FALSE ("element") FALSE ("element") FALSE ("element") TRUE ("element") TRUE ("element")] -> w373
              tunnel: [w623 TRUE ("element") TRUE ("element") FALSE ("element") FALSE ("element") FALSE ("element") FALSE ("element")] -> w372
              tunnel: [w624 FALSE ("element") FALSE ("element") TRUE ("element") TRUE ("element") TRUE ("element") TRUE ("element")] -> w371
              tunnel: [w622 FALSE ("element") FALSE ("element") TRUE ("element") TRUE ("element") FALSE ("element") FALSE ("element")] -> w365
              tunnel: [w625 FALSE ("element") FALSE ("element") TRUE ("element") TRUE ("element") FALSE ("element") FALSE ("element")] -> w370
              tunnel: [w621 FALSE ("element") FALSE ("element") FALSE ("element") FALSE ("element") TRUE ("element") TRUE ("element")] -> w343
              tunnel: [w626 TRUE ("element") TRUE ("element") TRUE ("element") TRUE ("element") FALSE ("element") FALSE ("element")] -> w369
              tunnel: [w619 FALSE ("element") FALSE ("element") FALSE ("element") FALSE ("element") TRUE ("element") TRUE ("element")] -> w368
              tunnel: [w618 30.0 70.0 30.0 70.0 0.0 0.0] -> w336
              tunnel: [w616 0.0 0.0 0.0 0.0 1.0 5.0] -> w335
              tunnel: [w617 0.0 0.0 0.0 0.0 15.0 15.0] -> w333
              frame 0, Default {
                w632 = ""
                # "Manual Control Test Parameters"
                n324 = local read "MC Instrumentation"() -> (w633:T4)
                n325 = Unbundle By Name(w633) -> ("SV1"=w630:bool, "SV2"=w629:bool, "SV3"=w628:bool, "SV4"=w627:bool, "SV5"=w620:bool, "SV6"=w623:bool, "SV7"=w624:bool, "SV8"=w622:bool, "SV9"=w625:bool, "M1"=w621:bool, "MP1"=w626:bool, "MP2"=w619:bool, "Motor Speed:"=w617:dbl, "CV1 Flow Rate:"=w616:dbl, "CV2 Flow Rate:"=w618:dbl)
                n326 = local read "MC Fields"() -> (w634:T3)
                n327 = Unbundle By Name(w634) -> ("MC Test Length"=w635:enum32{"Run Continuously", "Run for:"})
                n328 = case shown="\"Run Continuously\", Default" w635 {
                  tunnel: [2100000000 w637] -> w631
                  frame "Run Continuously", Default {
                  }
                  frame "Run for:" {
                    n329 = local read "MC Fields"() -> (w638:T3)
                    n330 = Unbundle By Name(w638) -> ("Test Duration"=w637:i64)
                  }
                }
              }
              frame 1 {
                # "Inhalation 30LPM Test Parameters"
                n331 = property on="Test Status:" class="Str"("Text.Scroll Position"=999) -> ()  [unwired: 2 in, 2 out]
                n332 = Concatenate Strings("Inhalation 30LPM initialising...", "\r\n") -> (w655:string)
                n333 = local read "Test Length"() -> (w639:i32)
              }
              frame 2 {
                # "Inhalation 70LPM Test Parameters"
                n334 = property on="Test Status:" class="Str"("Text.Scroll Position"=999) -> ()  [unwired: 2 in, 2 out]
                n335 = local read "Test Status:"() -> (w678:string)
                n336 = local read "Test Length"() -> (w660:i32)
                n337 = Concatenate Strings(w678, "Inhalation 70LPM test initialising...", "\r\n") -> (w676:string)
              }
              frame 3 {
                # "Exhalation 30LPM Test Parameters"
                n338 = property on="Test Status:" class="Str"("Text.Scroll Position"=999) -> ()  [unwired: 2 in, 2 out]
                n339 = local read "Test Status:"() -> (w700:string)
                n340 = local read "Test Length"() -> (w682:i32)
                n341 = Concatenate Strings(w700, "Exhalation 30LPM initialising...", "\r\n") -> (w698:string)
              }
              frame 4 {
                # "Exhalation 70LPM Test Parameters"
                n342 = property on="Test Status:" class="Str"("Text.Scroll Position"=999) -> ()  [unwired: 2 in, 2 out]
                n343 = local read "Test Status:"() -> (w722:string)
                n344 = local read "Test Length"() -> (w704:i32)
                n345 = Concatenate Strings(w722, "Exhalation 70LPM initialising...", "\r\n") -> (w720:string)
              }
              frame 5 {
                # "Breathing 15kft Test Parameters"
                n346 = property on="Test Status:" class="Str"("Text.Scroll Position"=999) -> ()  [unwired: 2 in, 2 out]
                n347 = local read "Test Status:"() -> (w744:string)
                n348 = local read "Test Length"() -> (w726:i32)
                n349 = Concatenate Strings(w744, "Breathing 15kft test initialising...", "\r\n") -> (w742:string)
              }
              frame 6 {
                # "Breathing 40kft Test Parameters"
                n350 = property on="Test Status:" class="Str"("Text.Scroll Position"=999) -> ()  [unwired: 2 in, 2 out]
                n351 = local read "Test Status:"() -> (w766:string)
                n352 = local read "Test Length"() -> (w748:i32)
                n353 = Concatenate Strings(w766, "Breathing 40kft test initialising...", "\r\n") -> (w764:string)
              }
            }
            n354 = local read "Test Buffer Duration"() -> (w342:i32)
            n355 = Add(x=w342, y=w341) -> (x+y=w340:i64)
            n356 = Build Array(w377, w376, w375, w374, w373, w372, w371, w365, w370, w343, w369, w368) -> (w367:bool[])
            n357 = Array Size(array=w367) -> (size(s)=w366:i32)
            n358 = call "Actuator Calculations.vi"("CV2 Flow Rate:"=w336, "CV1 Flow Rate:"=w335) -> ("CV2 Voltage"=w338:dbl, "CV1 Voltage"=w337:dbl)  [unwired: 8 in]
            n359 = for {
              N: w366 -> [_]
              tunnel: w367 -> [w394] mode=indexing
              tunnel: [w391] -> w364
              tunnel: [w390] -> w363
              tunnel: w325 -> [w387]
              tunnel: w324 -> [w386]
              i -> [w395]
              # "Relay Control"
              n360 = call "Relay Command Generator.vi"("Relay"=w395, "On/Off"=w394) -> ("Generated Command"=w393:string)  [unwired: 8 in]
              n361 = Concatenate Strings(w393, "\n" ("string")) -> (w389:string)
              n362 = VISA Write(VISA resource name=w386, write buffer=w389, error in (no error)=w387) -> (VISA resource name out=w390:refnum<visa-resource-name>, error out=w391:errorcluster)  [unwired: 1 out]
              n363 = Wait (ms)(milliseconds to wait=u32 20) -> ()  [unwired: 1 out]
            }
            n364 = local write "Total Test Time"(w340) -> ()
            n365 = local write "Test Duration"(w341) -> ()
            n366 = local write "Test Status:"(w378) -> ()
            n367 = local write "Current Test"(w379) -> ()
            n368 = local write "Motor Control"(w343) -> ()
            n369 = local write "Minute Volume"(w333) -> ()
            n370 = local write "CV1 Voltage"(w337) -> ()
            n371 = local write "CV2 Voltage"(w338) -> ()
            n372 = local write "In Progress"(FALSE ("In Progress")) -> ()
          }
          frame True {
          }
        }
      }
      n373 = for {
        N: 10 -> [_]
        tunnel: w272 -> [w295]
        tunnel: w271 -> [w294]
        tunnel: [w293] -> w208
        tunnel: [w292] -> w207
        n374 = Concatenate Strings("\":FE0F00000010020000E1\"" ("write buffer"), "\n" ("string")) -> (w291:string)
        n375 = VISA Write(VISA resource name=w294, write buffer=w291, error in (no error)=w295) -> (VISA resource name out=w292:refnum<visa-resource-name>, error out=w293:errorcluster)  [unwired: 1 out]
      }
      n376 = local write "Reference Voltage"(w211) -> ()
      n377 = call <vilib>:"DAQmx Stop Task.vi"("task/channels in"=w284, "error in"=w283) -> ("task out"=w282:refnum<k21>, "error out"=w281:errorcluster)  [unwired: 12 in]
      n378 = call <vilib>:"DAQmx Stop Task.vi"("task/channels in"=w268, "error in"=w267) -> ("task out"=w270:refnum<k21>, "error out"=w269:errorcluster)  [unwired: 12 in]
      n379 = call <vilib>:"DAQmx Stop Task.vi"("task/channels in"=w248, "error in"=w247) -> ("task out"=w258:refnum<k21>, "error out"=w259:errorcluster)  [unwired: 12 in]
      n380 = call <vilib>:"DAQmx Stop Task.vi"("task/channels in"=w231, "error in"=w232) -> ("task out"=w224:refnum<k21>, "error out"=w223:errorcluster)  [unwired: 12 in]
      n381 = call <vilib>:"DAQmx Clear Task.vi"("task in"=w282, "error in"=w281) -> ("error out"=w263:errorcluster)  [unwired: 13 in]
      n382 = call <vilib>:"DAQmx Clear Task.vi"("task in"=w270, "error in"=w269) -> ("error out"=w265:errorcluster)  [unwired: 13 in]
      n383 = call <vilib>:"DAQmx Clear Task.vi"("task in"=w258, "error in"=w259) -> ("error out"=w260:errorcluster)  [unwired: 13 in]
      n384 = call <vilib>:"DAQmx Clear Task.vi"("task in"=w224, "error in"=w223) -> ("error out"=w222:errorcluster)  [unwired: 13 in]
      n385 = call <vilib>:"Simple Error Handler.vi"("type of dialog (OK msg:1)"=w262, "error in (no error)"=w263) -> ()  [unwired: 3 in, 5 out]
      n386 = call <vilib>:"Simple Error Handler.vi"("type of dialog (OK msg:1)"=w264, "error in (no error)"=w265) -> ()  [unwired: 3 in, 5 out]
      n387 = call <vilib>:"Simple Error Handler.vi"("type of dialog (OK msg:1)"=w261, "error in (no error)"=w260) -> ()  [unwired: 3 in, 5 out]
      n388 = call <vilib>:"Simple Error Handler.vi"("type of dialog (OK msg:1)"=w221, "error in (no error)"=w222) -> ()  [unwired: 3 in, 5 out]
      n389 = VISA Flush I/O Buffer(VISA resource name=w207, error in (no error)=w208) -> (VISA resource name out=w210:refnum<visa-resource-name>, error out=w209:errorcluster)  [unwired: 1 in]
    }
  }
  n390 = case "Test Exit" shown="True" w39 {
    tunnel: [FALSE w790] -> w37
    frame False {
    }
    frame True {
      w789 = FALSE
      n391 = local read "Stop Test"() -> (w792:bool)
      n392 = property on="Test Status:" class="Str"("Text.Scroll Position"=999) -> ()  [unwired: 2 in, 2 out]
      n393 = case "Exit Type" shown="True" w792 {
        frame False {
          n394 = local read "Test Status:"() -> (w793:string)
          n395 = Concatenate Strings(w793, "All tests complete") -> (w794:string)
          n396 = local write "Test Status:"(w794) -> ()
        }
        frame True {
          n397 = local read "Test Status:"() -> (w797:string)
          n398 = Concatenate Strings(w797, "Testing Cancelled") -> (w798:string)
          n399 = local write "Test Status:"(w798) -> ()
        }
      }
      n400 = local read "Is PAT Test?"() -> (w790:bool)
      n401 = local write "Start Custom Test"(w789) -> ()
      n402 = local write "Start PAT Test"(w789) -> ()
      n403 = local write "Test Begin"(w789) -> ()
      n404 = local write "Motor Control"(w789) -> ()
    }
  }
  n405 = VISA Close(VISA resource name=w26, error in (no error)=w5) -> (error out=w1:errorcluster)
  n406 = call <vilib>:"Simple Error Handler.vi"("error in (no error)"=w1) -> ()  [unwired: 1 in, 8 out]
  n407 = case "Save Report" shown="True" w37 {
    frame False {
    }
    frame True {
      # "Save report"
      # "Report Title"
      # "Collect data headings for report"
      # "Collect data for report"
      n408 = local read "PAT Test Readings"() -> (w839:T1)
      n409 = local read "PAT Test Fields"() -> (w840:T2)
      n410 = property on="Test Date:" class="Str"() -> ("Label.Text"=w811:string)  [unwired: 2 in, 2 out]
      n411 = property on="Test Time:" class="Str"() -> ("Label.Text"=w810:string)  [unwired: 2 in, 2 out]
      n412 = property on="Operator:" class="Str"() -> ("Label.Text"=w809:string)  [unwired: 2 in, 2 out]
      n413 = property on="Pull Test Date:" class="Str"() -> ("Label.Text"=w808:string)  [unwired: 2 in, 2 out]
      n414 = property on="Manufacture Date:" class="Str"() -> ("Label.Text"=w807:string)  [unwired: 2 in, 2 out]
      n415 = property on="Cure Date:" class="Str"() -> ("Label.Text"=w806:string)  [unwired: 2 in, 2 out]
      n416 = property on="Production Order No.:" class="Str"() -> ("Label.Text"=w847:string)  [unwired: 2 in, 2 out]
      n417 = property on="Production Lot:" class="Str"() -> ("Label.Text"=w848:string)  [unwired: 2 in, 2 out]
      n418 = property on="No. Masks in Lot:" class="Str"() -> ("Label.Text"=w849:string)  [unwired: 2 in, 2 out]
      n419 = property on="Comments:" class="Str"() -> ("Label.Text"=w850:string)  [unwired: 2 in, 2 out]
      n420 = property on="F2 Leakage" class="DigNum (strict)"() -> ("Label.Text"=w822:string)  [unwired: 2 in, 2 out]
      n421 = property on="Ambient Humidity:" class="DigNum (strict)"() -> ("Label.Text"=w834:string)  [unwired: 2 in, 2 out]
      n422 = property on="Ambient Pressure:" class="DigNum (strict)"() -> ("Label.Text"=w833:string)  [unwired: 2 in, 2 out]
      n423 = property on="Ambient Temp.:" class="DigNum (strict)"() -> ("Label.Text"=w832:string)  [unwired: 2 in, 2 out]
      n424 = Unbundle By Name(w840) -> ("Test Date:"=w813:string, "Test Time:"=w821:string, "Operator:"=w820:string, "Pull Test Date:"=w819:string, "Manufacture Date:"=w818:string, "Cure Date:"=w817:string, "Production Order No.:"=w816:string, "Production Lot:"=w812:string, "No. Masks in Lot:"=w815:string, "Comments:"=w814:string, "F2 Leakage"=w799:dbl)
      n425 = Unbundle By Name(w839) -> ("In30 M"=w805:dbl, "In70 M"=w804:dbl, "Ex30 M"=w803:dbl, "Ex70 M"=w802:dbl, "B15 M"=w801:dbl, "B40 M"=w800:dbl)
      n426 = property on="Inhalation 30lpm" class="Str"() -> ("Value"=w851:string)  [unwired: 2 in, 2 out]
      n427 = property on="Inhalation 70lpm" class="Str"() -> ("Value"=w838:string)  [unwired: 2 in, 2 out]
      n428 = property on="Exhalation 30lpm" class="Str"() -> ("Value"=w823:string)  [unwired: 2 in, 2 out]
      n429 = property on="Exhalation 70lpm" class="Str"() -> ("Value"=w837:string)  [unwired: 2 in, 2 out]
      n430 = property on="Breathing 15kft" class="Str"() -> ("Value"=w836:string)  [unwired: 2 in, 2 out]
      n431 = property on="Breathing 40kft" class="Str"() -> ("Value"=w835:string)  [unwired: 2 in, 2 out]
      n432 = property on="Ambient Humidity:" class="DigNum (strict)"() -> ("Value"=w824:dbl)  [unwired: 2 in, 2 out]
      n433 = property on="Ambient Pressure:" class="DigNum (strict)"() -> ("Value"=w830:dbl)  [unwired: 2 in, 2 out]
      n434 = property on="Ambient Temp.:" class="DigNum (strict)"() -> ("Value"=w829:dbl)  [unwired: 2 in, 2 out]
      n435 = Build Array(w811, w810, w809, w808, w807, w806, w847, w848, w849, w850, w851, w838, w823, w837, w836, w835, w822, w834, w833, w832) -> (w842:string[])
      n436 = Build Array(w805, w804, w803, w802, w801, w800, w799, w824, w830, w829) -> (w831:dbl[])
      n437 = Number To Fractional String(number=w831, precision (6)=3) -> (F-format string=w827:string[])  [unwired: 2 in]
      n438 = Build Array(w813, w821, w820, w819, w818, w817, w816, w812, w815, w814) -> (w828:string[])
      n439 = Insert Into Array(array=w828, new element=w827) -> (w825:string[])  [unwired: 1 in]
      n440 = local read "Results File Location:"() -> (w843:path)
      n441 = Concatenate Strings(w813, " Testing - ", w812) -> (w841:string)
      n442 = call "Save Report SubVI.vi"("File Name"=w841, "error in (no error)"="error in (no error)", "Fields"=w842, "Inputs"=w825, "Results File Location:"=w843) -> ("error out"=→"error out":errorcluster)  [unwired: 6 in]
    }
  }
